vi "AD7714 Sample.vi"(9 "Channel":i16, 11 "I/O Cluster In":T1) -> (1 "Data":u32 format="%b", 2 "Raw Data Response (MSB)":bool[](array[boolean]), 3 "I/O Cluster Out":T1)   [LabVIEW 2018, in "jmslib.lvlib"]
uses:
  jmslib.lvlib
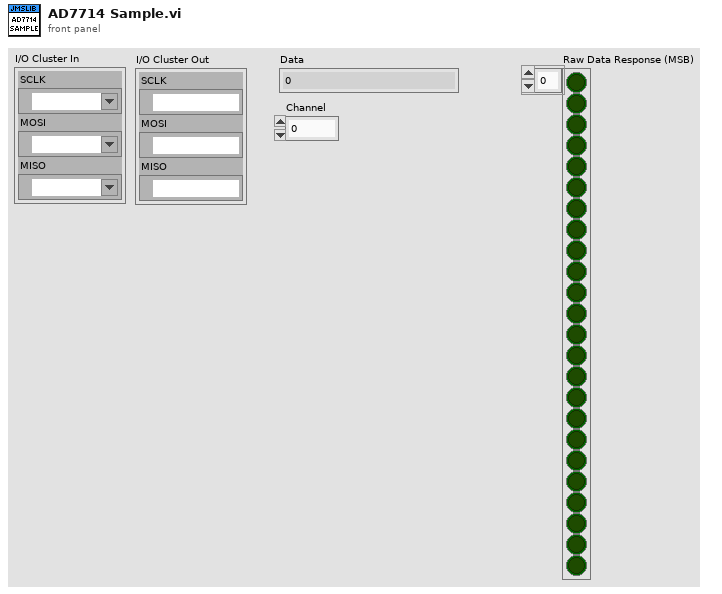
[diagram p1: front panel]
types:
  T1 = cluster{"SCLK":refnum<k21>, "MOSI":refnum<k21>, "MISO":refnum<k21>}
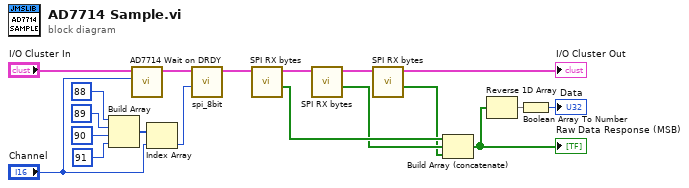
[diagram p0: block diagram]
diagram:
  n1 = Build Array(i8 88, i8 89, i8 90, i8 91) -> (w14:i8[])
  n2 = call "AD7714 Wait on DRDY.vi"("Channel"="Channel", "I/O Cluster In"="I/O Cluster In") -> ("I/O Cluster Out"=w11:T1)  [unwired: 7 in, 2 out]
  n3 = Index Array(array=w14, index="Channel") -> (element=w2:i8)
  n4 = call "spi_8bit.vi"("Hex"=w2, "I/O Cluster In"=w11) -> ("I/O Cluster Out"=w10:T1)  [unwired: 9 in]
  n5 = call "SPI RX bytes.vi"("I/O Cluster In"=w10) -> ("Output Byte"=w7:bool[], "I/O Cluster Out"=w9:T1)  [unwired: 9 in]
  n6 = call "SPI RX bytes.vi"("I/O Cluster In"=w9) -> ("Output Byte"=w6:bool[], "I/O Cluster Out"=w8:T1)  [unwired: 9 in]
  n7 = call "SPI RX bytes.vi"("I/O Cluster In"=w8) -> ("Output Byte"=w5:bool[], "I/O Cluster Out"=→"I/O Cluster Out":T1)  [unwired: 9 in]
  n8 = Build Array (concatenate)(w7, w6, w5) -> (w4:bool[])
  "Raw Data Response (MSB)" <- w4
  n9 = Reverse 1D Array(array=w4) -> (reversed array=w3:bool[])
  n10 = Boolean Array To Number(Boolean array=w3) -> (number=→"Data":u32)
